vi "切换出图为TNR.vi"(8 "error in":errorcluster) -> (0 "error out":errorcluster, 3 "return":i32)   [LabVIEW 2016]
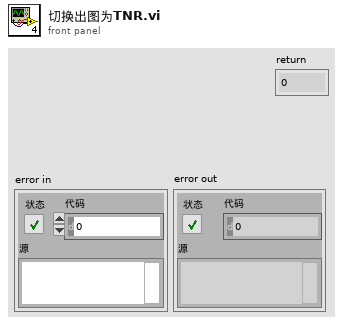
[diagram p1: front panel]
types:
  T1 = cluster{"byCmdType":u8, "bySubCmd":u8, "byPara":u8, "byAddr_h":u8, "byAddr_l":u8, "byAddr_ll":u8, "byLen_h":u8, "byLen_l":u8}
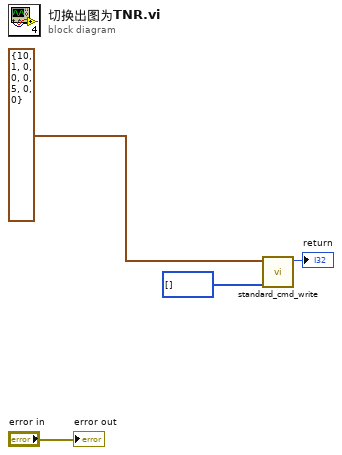
[diagram p0: block diagram]
diagram:
  n1 = call "standard_cmd_write.vi"("data"=u8[] [], "cmd_std_header_t"=T1 {"byCmdType"=10, "bySubCmd"=1, "byPara"=0, "byAddr_h"=0, "byAddr_l"=0, "byAddr_ll"=5, "byLen_h"=0, "byLen_l"=0}) -> ("return"=→"return":i32)  [unwired: 8 in, 1 out]
  "error out" <- "error in"
